vi "createGObject.vi"(8 "error in (no error)":errorcluster, 10 "GObjectSelection":T1, 11 "GObjectFactory in":refnum<class "GObjectFactory.lvclass">) -> (0 "error out":errorcluster, 2 "GObject":refnum<class "GObject.lvclass">, 3 "GObjectFactory out":refnum<class "GObjectFactory.lvclass">)   [LabVIEW 2016, in "GObjectFactory.lvclass"]
uses:
  GObjectFactory.lvclass
  Typedefs/GObjectSelection.ctl
  GObject/GObject.lvclass
  GObjects/DefaultDiagramObject/DefaultDiagramObject.lvclass
  home/plotz/lsst_ts/ct_tools/GObject/GObject.lvclass
  GObjects/CaseStructure/CaseStructure.lvclass
  GObjects/ClusterConstant/ClusterConstant.lvclass
  GObjects/EnumConstant/EnumConstant.lvclass
  GObjects/EventStructure/EventStructure.lvclass
  GObjects/FlatSequence/FlatSequence.lvclass
  GObjects/ForLoop/ForLoop.lvclass
  GObjects/WhileLoop/WhileLoop.lvclass
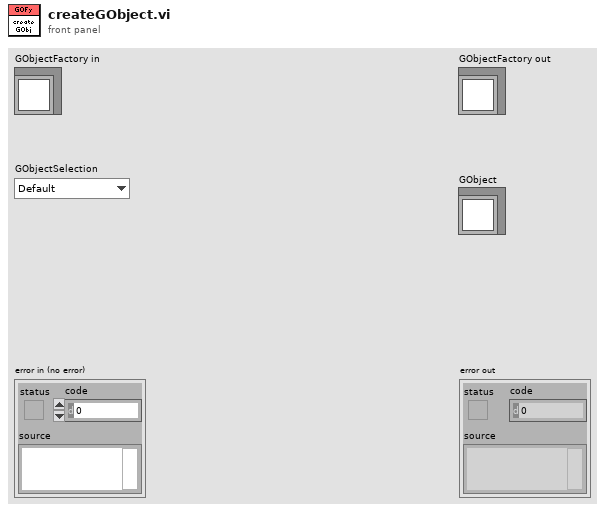
[diagram p1: front panel]
types:
  T1 = typedef "GObjectSelection.ctl" = enum16{"Default", "CaseStructure", "ClusterConstant", "EnumConstant", "EventStructure", "FlatSequence", "ForLoop", "WhileLoop"}
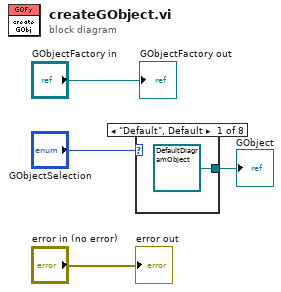
[diagram p0: block diagram]
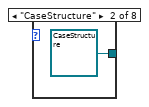
[diagram p2: hidden frame]
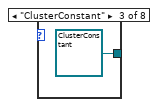
[diagram p3: hidden frame]
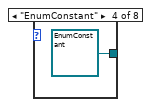
[diagram p4: hidden frame]
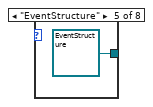
[diagram p5: hidden frame]
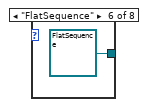
[diagram p6: hidden frame]
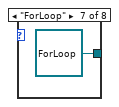
[diagram p7: hidden frame]
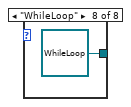
[diagram p8: hidden frame]
diagram:
  n1 = case shown="\"Default\", Default" "GObjectSelection" {
    tunnel: [refnum<class "DefaultDiagramObject.lvclass"> refnum ("DefaultDiagramObject.lvclass") refnum<class "CaseStructure.lvclass"> refnum ("CaseStructure.lvclass") refnum<class "ClusterConstant.lvclass"> refnum ("ClusterConstant.lvclass") refnum<class "EnumConstant.lvclass"> refnum ("EnumConstant.lvclass") refnum<class "EventStructure.lvclass"> refnum ("EventStructure.lvclass") refnum<class "FlatSequence.lvclass"> refnum ("FlatSequence.lvclass") refnum<class "ForLoop.lvclass"> refnum ("ForLoop.lvclass") refnum<class "WhileLoop.lvclass"> refnum ("WhileLoop.lvclass")] -> w2
    frame "Default", Default {
    }
    frame "CaseStructure" {
    }
    frame "ClusterConstant" {
    }
    frame "EnumConstant" {
    }
    frame "EventStructure" {
    }
    frame "FlatSequence" {
    }
    frame "ForLoop" {
    }
    frame "WhileLoop" {
    }
  }
  "GObject" <- w2
  "error out" <- "error in (no error)"
  "GObjectFactory out" <- "GObjectFactory in"
